vi "ProyectoBioCuinique Alpha 1.0.vi"() -> ()   [LabVIEW 2021]
uses:
  <vilib>/Utility/NIReport.llb/Report Type.ctl
  <extravilib>/ChannelInstances/Tag-bool/Read With Abort.vi
  <extravilib>/ChannelInstances/Tag-bool/Write With Abort.vi
  <vilib>/Instr/_visa.llb/VISA Configure Serial Port (Instr).vi
  <vilib>/MakerHub/LINX/Public/Utilities/Open Serial.vi
  <extravilib>/ChannelInstances/Tag-bool/Instantiate.vi
  <vilib>/addons/_office/excel.llb/Excel Easy Table (str).vi
  <extravilib>/ChannelInstances/Tag-bool/EndpointRead.vi
  <extravilib>/ChannelInstances/Tag-bool/Endpoint.vi
  <vilib>/Utility/NIReport.llb/NI_report.lvclass
  <vilib>/LabVIEW Interface for Arduino/LabVIEW Interface for Arduino.lvlib
  <vilib>/MakerHub/LINX/LMH-LINX.lvlib
  <vilib>/Utility/NIReport.llb/NI_ReportGenerationCore.lvlib
  <vilib>/addons/_office/NI_ReportGenerationToolkit.lvlib
  <vilib>/Utility/NIReport.llb/Excel/NI_Excel.lvclass
  <vilib>/MakerHub/LINX/Public/Sensors/Distance/Ultrasonic/Ultrasonic.lvlib
  <extravilib>/ChannelInstances/Tag-bool.lvlib
panel:
  in  "Temperatura":dbl(slide) scale=0.0..100.0
  in  "Iluminidad":dbl(knob) scale=0.0..10.0
  in  "template (empty)":path
  in  "Pin Bomba 1":u8
  in  "Pin Valvula 1":u8
  in  "Pin Valvula 2":u8
  out "HUMEDAD 2":dbl
  in  "VISA resource name":refnum<visa-resource-name>
  out "TEMPERATURA":dbl
  out "HUMEDAD":dbl(knob) scale=0.0..255.0
  out "Centimeters":dbl
  out "Slide":dbl(slide) scale=0.0..500.0
  out "BOMBA (11)":bool
  in  "Boolean 4":bool
  out "VALVULA (6)":bool
  in  "Boolean":bool
  out "VALVULA (5)":bool
  in  "stop":bool
  in  "VISA resource":refnum<visa-resource-name>
  # "VÁLVULA 1"
  # "BOMBA DE AGUA"
  # "VÁLVULA 2"
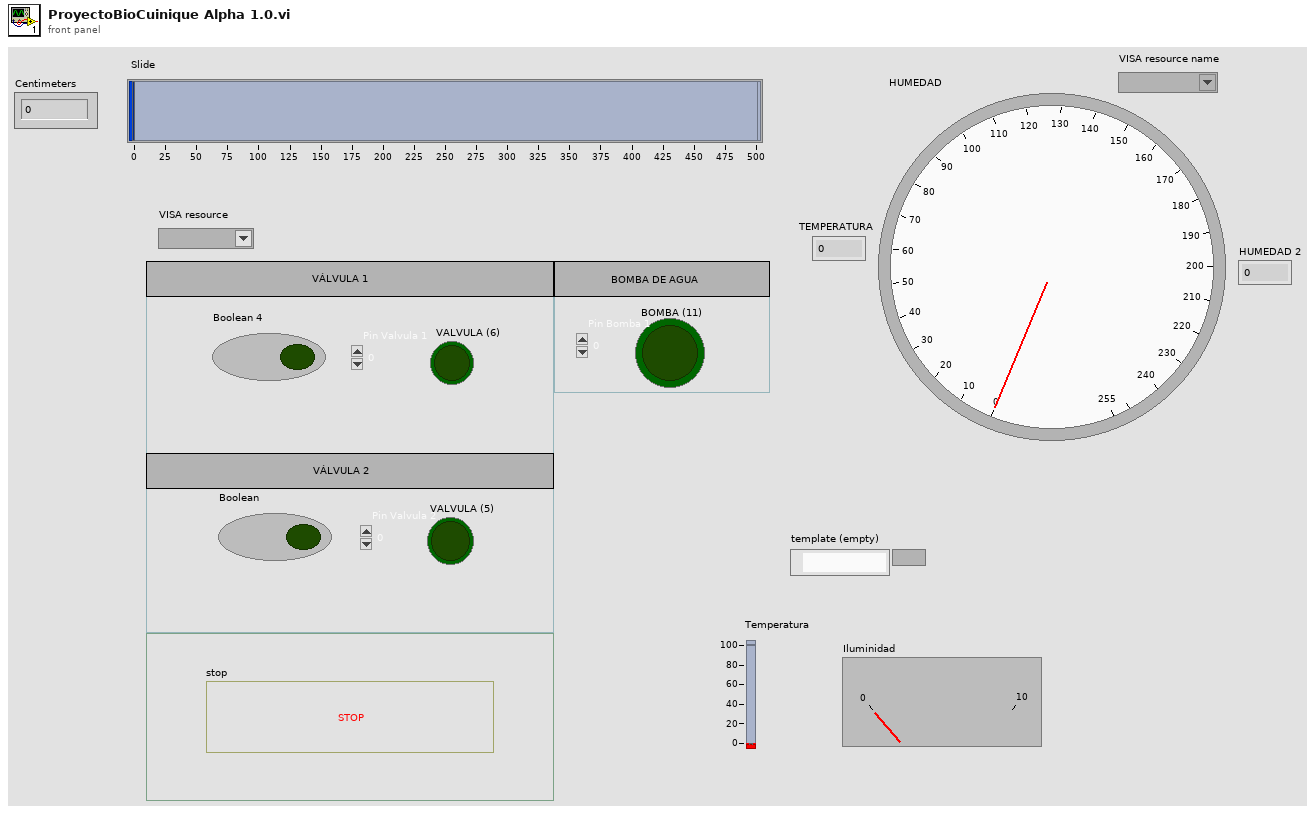
[diagram p1: front panel]
types:
  T1 = typedef "NI_ReportGenerationCore.lvlib/Report Type.ctl" = enum16{"HTML", "Word", "Excel"}
  T2 = typedef "LabVIEW Interface for Arduino.lvlib/Arduino Resource.ctl" = cluster{"VISA resource":refnum<visa-resource-name>, "Board Type":T3, "Connection Type":enum8{"USB / Serial"}, "Bytes Per Packet (15)":u8}
  T3 = typedef "LabVIEW Interface for Arduino.lvlib/Board Type.ctl" = enum16{"Uno", "Dimuelanove w/Atmega 328", "Mega 2560"}
  T4 = typedef "LMH-LINX.lvlib/LINX Ref.ctl" = cluster{"IO":T5, "Interface":T6, "LINX Device Config":T7}
  T5 = typedef "LMH-LINX.lvlib/Platform.ctl" = enum16{"Remote", "Local"}
  T6 = typedef "LMH-LINX.lvlib/Interface.ctl" = enum16{"Serial", "TCP"}
  T7 = typedef "LMH-LINX.lvlib/Device.lvlib/LINX Device Config.ctl" = cluster{"Interface":T6, "COM Port":refnum<visa-resource-name>, "TCP Configuration":T8, "Device Family":u8, "Device ID":u8, "Device Name":string, "TCP Ref":refnum<k5>, "Channels":T9}
  T8 = typedef "LMH-LINX.lvlib/Device.lvlib/TCP Config.ctl" = cluster{"IP Address":string, "Port":u16}
  T9 = typedef "LMH-LINX.lvlib/Channels.ctl" = cluster{"DI":u8[], "DO":u8[], "AI":u8[], "AO":u8[], "PWM":u8[], "QE":u8[], "UART":u8[], "I2C 2":u8[], "SPI":u8[], "CAN":u8[], "Servo":u8[], "AI Ref (V)":dbl, "AI Resolution (Bits)":u8, "AO Ref (V)":dbl, "AO Resolution (Bits)":u8}
  T10 = typedef "Tag-bool.lvlib/))Channel.ctl" = refnum<queue>
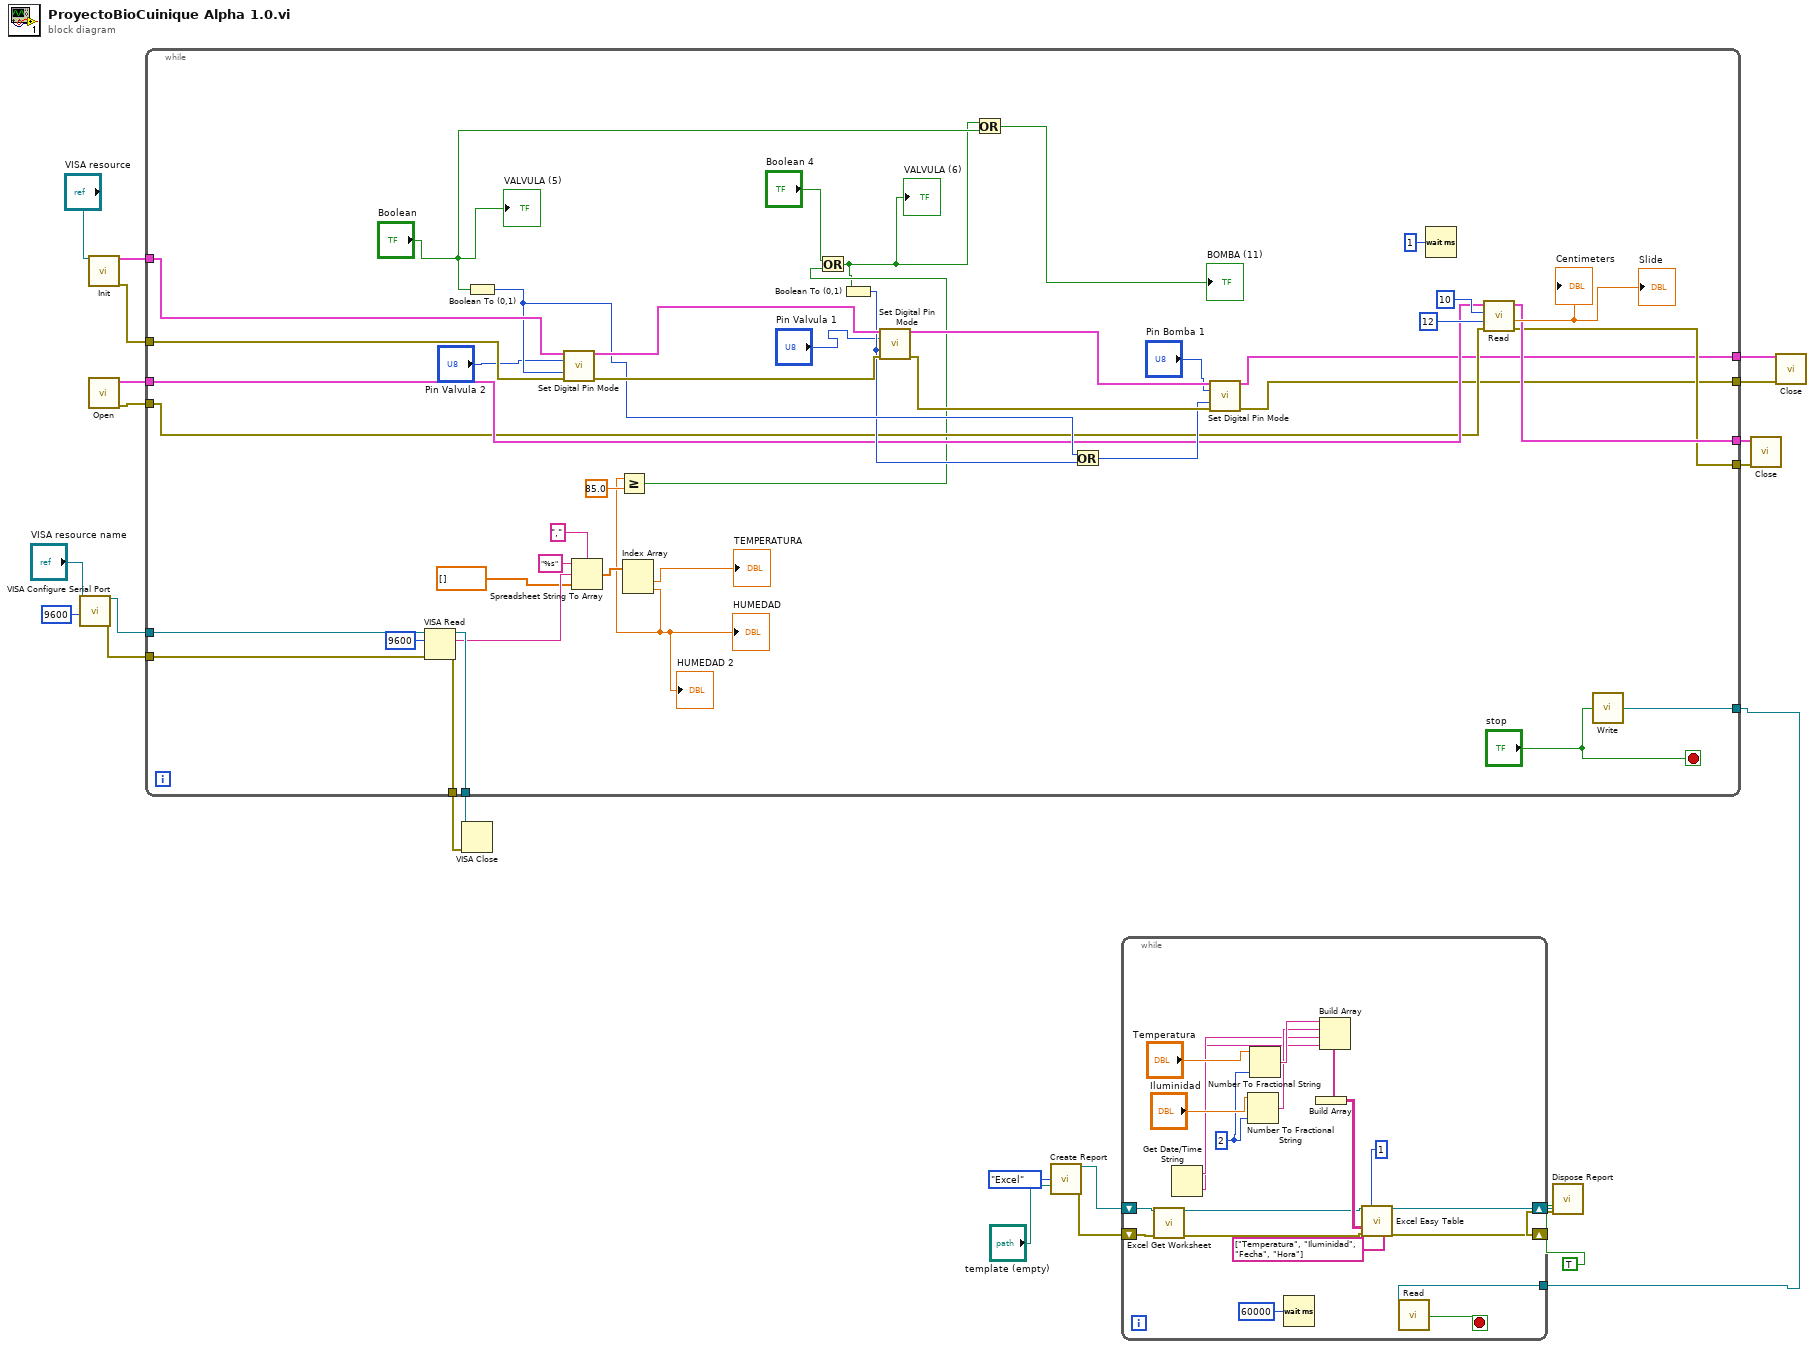
[diagram p0: block diagram]
diagram:
  n1 = call-poly "VISA Configure Serial Port"("VISA resource name"="VISA resource name", "baud rate (9600)"=u32 9600) -> ("VISA resource name out"=w14:refnum<visa-resource-name>, "error out"=w11:errorcluster)  [unwired: 12 in]
  n2 = call <vilib>:"Init.vi"("VISA resource"="VISA resource") -> ("Arduino Resource"=w22:T2, "error out"=w21:errorcluster)  [unwired: 17 in]
  n3 = call-poly <vilib>:"Open.vi"() -> ("Error Out"=w20:errorcluster, "LINX Resource"=w19:T4)  [unwired: 9 in, 1 out]
  n4 = while {
    tunnel: w22 -> [w65]
    tunnel: w21 -> [w64]
    tunnel: w20 -> [w50]
    tunnel: w19 -> [w51]
    tunnel: [w49] -> w18
    tunnel: [w48] -> w17
    tunnel: [w47] -> w16
    tunnel: [w46] -> w15
    tunnel: w14 -> [w45]
    tunnel: [w44] -> w13
    tunnel: [w43] -> w12
    tunnel: w11 -> [w42]
    tunnel: [w24] -> w1
    stop <- "stop" stop-if-true
    n5 = VISA Read(VISA resource name=w45, byte count=u32 9600, error in (no error)=w42) -> (VISA resource name out=w43:refnum<visa-resource-name>, read buffer=w41:string, error out=w44:errorcluster)  [unwired: 1 out]
    n6 = Boolean To (0,1)(Boolean="Boolean") -> (0, 1=w59:i16)
    n7 = call <vilib>:"Set Digital Pin Mode.vi"("Arduino Resource"=w65, "Digital I/O Pin"="Pin Valvula 2", "Pin Mode (Input)"=w59, "error in"=w64) -> ("Arduino Resource"=w63:T2, "error out"=w62:errorcluster)  [unwired: 10 in]
    n8 = Spreadsheet String To Array(delimiter (Tab)=",", format string="%s", spreadsheet string=w41, array type (2D Dbl)=dbl[] []) -> (array=w37:dbl[])
    n9 = Index Array(array=w37) -> (element #1=→"TEMPERATURA":dbl, element #2=w33:dbl)  [unwired: 2 in]
    "HUMEDAD" <- w33
    "HUMEDAD 2" <- w33
    n10 = Greater Or Equal?(x=w33, y=85.0) -> (x >= y?=w31:bool)
    n11 = Or(x="Boolean 4", y=w31) -> (x .or. y?=w29:bool)
    "VALVULA (6)" <- w29
    n12 = Boolean To (0,1)(Boolean=w29) -> (0, 1=w58:i16)
    n13 = call <vilib>:"Set Digital Pin Mode.vi"("Arduino Resource"=w63, "Digital I/O Pin"="Pin Valvula 1", "Pin Mode (Input)"=w58, "error in"=w62) -> ("Arduino Resource"=w60:T2, "error out"=w61:errorcluster)  [unwired: 10 in]
    n14 = Or(x=w29, y="Boolean") -> (x .or. y?=→"BOMBA (11)":bool)
    n15 = Or(x=w59, y=w58) -> (x .or. y?=w57:i16)
    n16 = call <vilib>:"Set Digital Pin Mode.vi"("Arduino Resource"=w60, "Digital I/O Pin"="Pin Bomba 1", "Pin Mode (Input)"=w57, "error in"=w61) -> ("Arduino Resource"=w47:T2, "error out"=w46:errorcluster)  [unwired: 10 in]
    n17 = Wait (ms)(milliseconds to wait=u32 1) -> ()  [unwired: 1 out]
    n18 = call <vilib>:"Read.vi"("Error In"=w50, "DO Channel"=u8 12, "DI Channel"=u8 10, "LINX Resource"=w51) -> ("Error Out"=w48:errorcluster, "Centimeters"=→"Centimeters" →"Slide":dbl, "LINX Resource"=w49:T4)  [unwired: 4 in, 1 out]
    n19 = call <extravilib>:"Write.vi"("element"="stop") -> ("channel"=w24:T10)  [unwired: 1 out]
    "VALVULA (5)" <- "Boolean"
  }
  n20 = VISA Close(VISA resource name=w12, error in (no error)=w13) -> ()  [unwired: 1 out]
  n21 = call <vilib>:"Create Report.vi"("report type"=Report_Type."Excel", "template (empty)"="template (empty)") -> ("report out"=w5:refnum<class "NI_report.lvclass">, "error out"=w6:errorcluster)  [unwired: 12 in]
  n22 = while {
    shift-right: [w71] -> w3
    shift-left: w6 -> [w76]
    shift-right: [w72] -> w4
    shift-left: w5 -> [w74]
    tunnel: w1 -> [w67]
    stop <- w66 stop-if-true
    w83 = i16 2 ("precision (6)")
    n23 = call <vilib>:"Excel Get Worksheet.vi"("report in"=w74, "error in (no error)"=w76) -> ("report out"=w73:refnum<class "NI_report.lvclass">, "error out"=w75:errorcluster)  [unwired: 12 in]
    n24 = Get Date/Time String() -> (date string=w80:string, time string=w79:string)  [unwired: 3 in]
    n25 = Number To Fractional String(number="Iluminidad", precision (6)=w83) -> (F-format string=w81:string)  [unwired: 2 in]
    n26 = Number To Fractional String(number="Temperatura", precision (6)=w83) -> (F-format string=w82:string)  [unwired: 2 in]
    n27 = Wait (ms)(milliseconds to wait=u32 60000) -> ()  [unwired: 1 out]
    n28 = Build Array(w82, w81, w80, w79) -> (w78:string[])
    n29 = Build Array(w78) -> (w77:string[][])
    n30 = call-poly <vilib>:"Excel Easy Table.vi"("report in"=w73, "iteration"=1, "text data"=w77, "error in (no error)"=w75, "column headers"=string[] ["Temperatura", "Iluminidad", "Fecha", "Hora"]) -> ("report out"=w72:refnum<class "NI_report.lvclass">, "error out"=w71:errorcluster)  [unwired: 6 in, 3 out]
    n31 = call <vilib>:"Read.vi"("channel"=w67) -> ("element"=w66:bool)  [unwired: 1 in, 1 out]
  }
  n32 = call-dynamic "Dispose Report.vi"("report in"=w4, "save changes? (F)"=TRUE, "error in (no error)"=w3) -> ()  [unwired: 12 in, 1 out]
  n33 = call <vilib>:"Close.vi"("Error In"=w17, "LINX Resource"=w18) -> ()  [unwired: 9 in, 1 out]
  n34 = call <vilib>:"Close.vi"("Arduino Resource"=w16, "error in"=w15) -> ()  [unwired: 13 in, 1 out]
